vi "UART Get.vi"(8 "error in (no error)":errorcluster, 11 "Command":string) -> (0 "error out":errorcluster, 3 "Returned String":string)   [LabVIEW 2013]
uses:
  filter wheel/Libraries/uart_library.dll
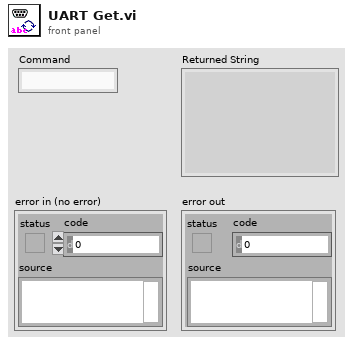
[diagram p1: front panel]
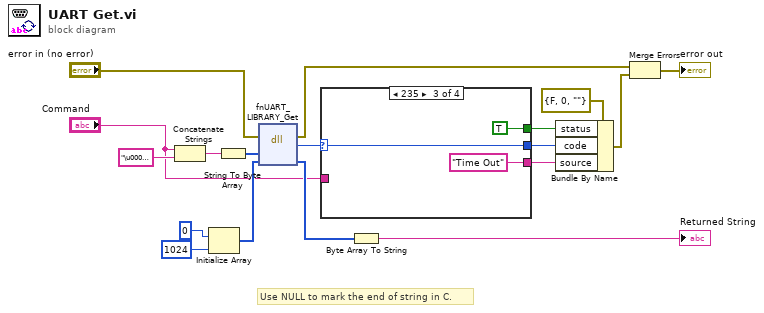
[diagram p0: block diagram]
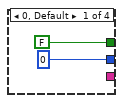
[diagram p2: hidden frame]
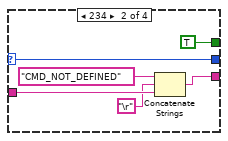
[diagram p3: hidden frame]
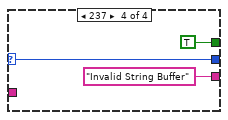
[diagram p4: hidden frame]
diagram:
  # "Use NULL to mark the end of string in C."
  n1 = Concatenate Strings("Command", "\u0000\u0000") -> (w17:string)
  n2 = Initialize Array(u8 0, 1024 ("dimension size")) -> (w10:u8[])
  n3 = String To Byte Array(string=w17) -> (unsigned byte array=w16:u8[])
  n4 = dll-call lib="E:/users/tba/work_project/FW102/trunk/LabVIEW/Libraries/uart_library.dll" fn="fnUART_LIBRARY_Get"(error in="error in (no error)", "Input Command"=w16, "Returned String"=w10) -> (error out=w4:errorcluster, "return type"=w15:i32, "Returned String"=w14:u8[])  [unwired: 3 in, 1 out]
  n5 = case shown="235" w15 {
    selector: w15 -> [_ w25 w27 w30]
    tunnel: [_ w21 "Time Out" "Invalid String Buffer"] -> w5
    tunnel: [FALSE TRUE TRUE TRUE] -> w7
    tunnel: [0 w25 w27 w30] -> w6
    tunnel: "Command" -> [_ w23 _ _]
    frame 0, Default {
    }
    frame 234 {
      n6 = Concatenate Strings("CMD_NOT_DEFINED", "\r", w23) -> (w21:string)
    }
    frame 235 {
    }
    frame 237 {
    }
  }
  n7 = Byte Array To String(unsigned byte array=w14) -> (string=→"Returned String":string)
  n8 = Bundle By Name(cluster=errorcluster {"status"=FALSE, "code"=0, "source"=""} ("error out"), "status"=w7, "code"=w6, "source"=w5) -> (w3:errorcluster)
  n9 = Merge Errors(w4, w3) -> (→"error out":errorcluster)
